vi "Init from PS.vi"(8 "error in (no error)":errorcluster, 11 "PS Control Actor in":refnum<class "PS Control Actor.lvclass">) -> (0 "error out":errorcluster, 3 "PS Control Actor out":refnum<class "PS Control Actor.lvclass">)   [LabVIEW 2021, in "PS Control Actor.lvlib" / "PS Control Actor.lvclass"]
uses:
  PS Control Actor.lvclass
  PS Driver/PS Driver.lvclass
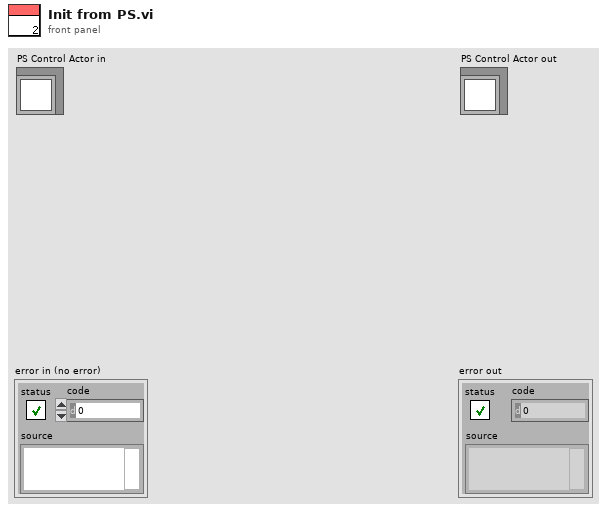
[diagram p1: front panel]
types:
  T1 = cluster{"User rate (A/sec)":dbl, "Last programmed rate (A/sec)":dbl, "Ramp status":enum16{"Hold", "Ramp to zero", "Ramp to setpoint"}, "Setpoint (A)":dbl}
  T2 = enum16{"Hold", "Ramp to zero", "Ramp to setpoint"}
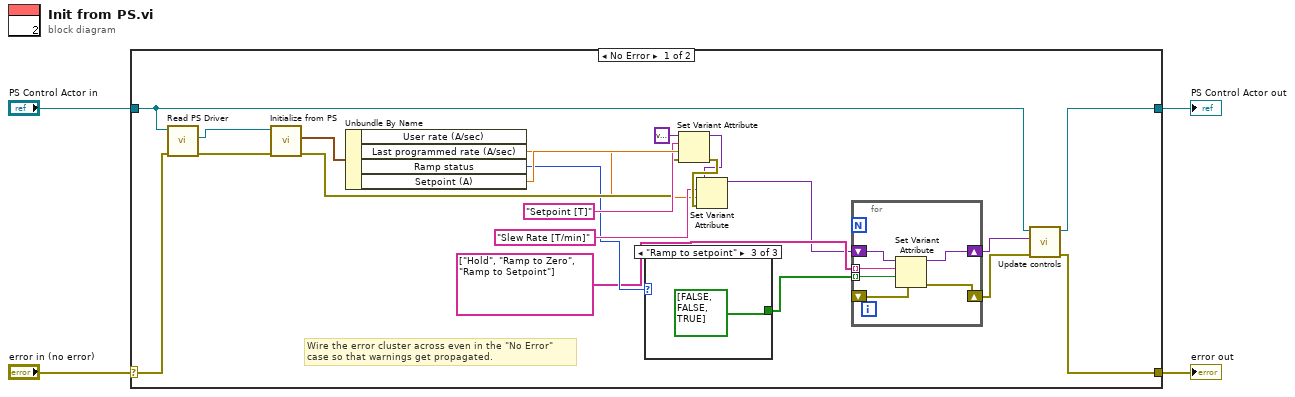
[diagram p0: block diagram]
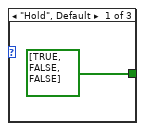
[diagram p2: hidden frame]
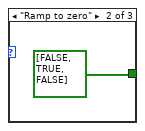
[diagram p3: hidden frame]
diagram:
  n1 = case shown="No Error" "error in (no error)" {
    selector: "error in (no error)" -> [w25 w36]
    tunnel: [w8 w36] -> w3
    tunnel: [w9 w35] -> w1
    tunnel: "PS Control Actor in" -> [w10 w35]
    frame No Error {
      # "Wire the error cluster across even in the \"No Error\"\ncase so that warnings get propagated."
      n2 = call-dynamic "Read PS Driver.vi"("error in (no error)"=w25, "PS Control Actor in"=w10) -> ("error out"=w24:errorcluster, "PS Driver.lvlib:PS Driver.lvclass"=w23:refnum<class "PS Driver.lvclass">)  [unwired: 7 in, 1 out]
      n3 = call-dynamic "Initialize from PS.vi"("error in (no error)"=w24, "PS Driver in"=w23) -> ("error out"=w18:errorcluster, "PS Values"=w22:T1)  [unwired: 7 in, 1 out]
      n4 = Unbundle By Name(w22) -> ("Last programmed rate (A/sec)"=w14:dbl, "Ramp status"=w13:T2, "Setpoint (A)"=w21:dbl)  [unwired: 1 out]
      n5 = case shown="\"Ramp to setpoint\"" w13 {
        tunnel: [bool[] [TRUE, FALSE, FALSE] bool[] [FALSE, TRUE, FALSE] bool[] [FALSE, FALSE, TRUE]] -> w12
        frame "Hold", Default {
        }
        frame "Ramp to zero" {
        }
        frame "Ramp to setpoint" {
        }
      }
      n6 = Set Variant Attribute(Variant=variant ("variant"), name="Setpoint [T]" ("Control Name"), value=w21, error in=w18) -> (Variant out=w16:variant, error out=w17:errorcluster)  [unwired: 1 out]
      n7 = Set Variant Attribute(Variant=w16, name="Slew Rate [T/min]" ("Control Name"), value=w14, error in=w17) -> (Variant out=w5:variant)  [unwired: 2 out]
      n8 = for {
        shift-right: [w32] -> w6
        shift-left: w5 -> [w33]
        shift-right: [w31] -> w7
        shift-left: _ -> [w34]
        tunnel: string[] ["Hold", "Ramp to Zero", "Ramp to Setpoint"] -> [w30] mode=indexing
        tunnel: w12 -> [w29] mode=indexing
        n9 = Set Variant Attribute(Variant=w33, name=w30, value=w29, error in=w34) -> (Variant out=w32:variant, error out=w31:errorcluster)  [unwired: 1 out]
      }
      n10 = call "Update controls.vi"("error in (no error)"=w7, "New control values"=w6, "PS Control Actor in"=w10) -> ("error out"=w8:errorcluster, "PS Control Actor out"=w9:refnum<class "PS Control Actor.lvclass">)  [unwired: 7 in]
    }
    frame Error {
    }
  }
  "error out" <- w3
  "PS Control Actor out" <- w1
